vi "CLSUIP_GetControlInformation.vi"(8 "error in (no error)":errorcluster, 11 "Ctl Refnum":refnum<vi>) -> (0 "error out":errorcluster, 2 "Control Information":T1, 3 "Ctl Refnum out":refnum<vi>)   [LabVIEW 2021, in "MemberVICreation.lvlib"]
uses:
  <resource>/Framework/Providers/LVClassLibrary/NewAccessors/MemberVICreation.lvlib
  <resource>/Framework/Providers/LVClassLibrary/NewAccessors/CLSUIP_ControlInformation.ctl
  <vilib>/Utility/miscctls.llb/LVPositionTypeDef.ctl
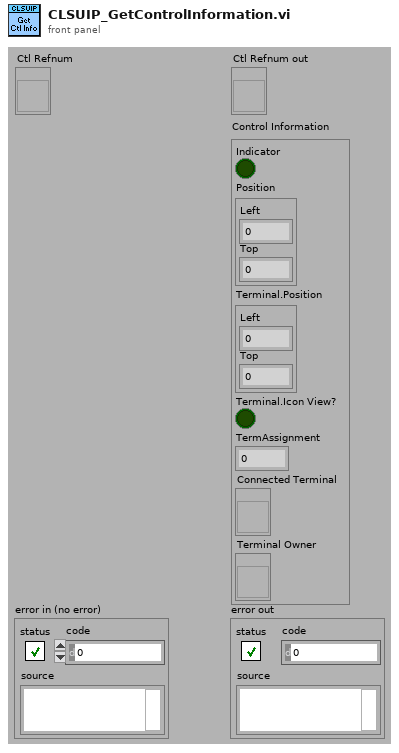
[diagram p1: front panel]
types:
  T1 = typedef "MemberVICreation.lvlib/CLSUIP_ControlInformation.ctl" = cluster{"Indicator":bool, "Position":T2, "Terminal.Position":T2, "Terminal.Icon View?":bool, "TermAssignment":i32, "Connected Terminal":refnum<vi>, "Terminal Owner":refnum<vi>}
  T2 = typedef "LVPositionTypeDef.ctl" = cluster{"Left":i32, "Top":i32}
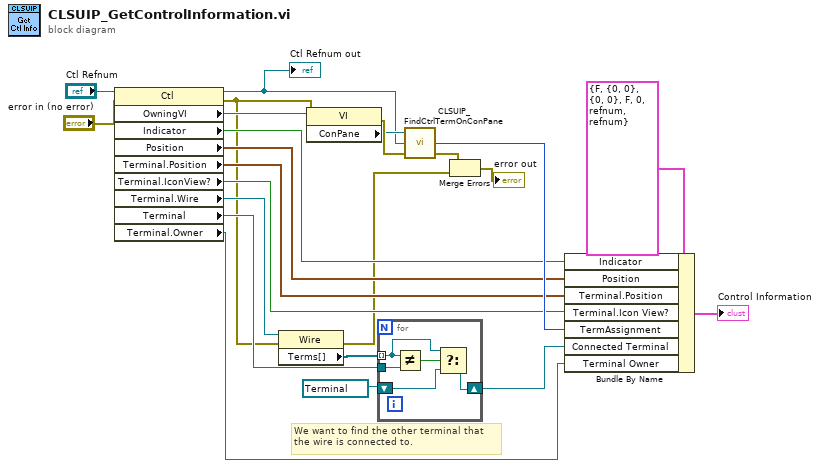
[diagram p0: block diagram]
diagram:
  # "We want to find the other terminal that\nthe wire is connected to."
  n1 = property class="Ctl"(reference="Ctl Refnum", error in="error in (no error)") -> (reference out=w11:refnum<vi>, error out=w5:errorcluster, "OwningVI"=w22:refnum<vi>, "Indicator"=w19:bool, "Position"=w18:T2, "Terminal.Position"=w17:T2, "Terminal.IconView?"=w16:bool, "Terminal.Wire"=w10:refnum<vi>, "Terminal"=w8:refnum<vi>, "Terminal.Owner"=w1:refnum<vi>)
  "Ctl Refnum out" <- w11
  n2 = property class="Wire"(reference=w10, error in=w5) -> (error out=w3:errorcluster, "Terms[]"=w9:refnum<vi>[])  [unwired: 1 out]
  n3 = property class="VI"(reference=w22, error in=w5) -> (error out=w14:errorcluster, "ConPane"=w12:refnum<vi>)  [unwired: 1 out]
  n4 = for {
    tunnel: w9 -> [w24] mode=indexing
    shift-right: [w25] -> w7
    shift-left: refnum<vi> refnum ("Connected Terminal") -> [w26]
    tunnel: w8 -> [w27]
    n5 = Not Equal?(x=w24, y=w27) -> (x != y?=w28:bool)
    n6 = Select(t=w24, s=w28, f=w26) -> (s? t:f=w25:refnum<vi>)
  }
  n7 = call <resource>:"CLSUIP_FindCtrlTermOnConPane.vi"("error in (no error)"=w14, "Ctl Refnum"=w11, "ConPane"=w12) -> ("error out"=w4:errorcluster, "Terminal Index"=w20:i32)  [unwired: 1 out]
  n8 = Merge Errors(w4, w3) -> (→"error out":errorcluster)
  n9 = Bundle By Name(cluster=T1 {"Indicator"=FALSE, "Position"={"Left"=0, "Top"=0}, "Terminal.Position"={"Left"=0, "Top"=0}, "Terminal.Icon View?"=FALSE, "TermAssignment"=0, "Connected Terminal"=refnum, "Terminal Owner"=refnum} ("Control Information"), "Indicator"=w19, "Position"=w18, "Terminal.Position"=w17, "Terminal.Icon View?"=w16, "TermAssignment"=w20, "Connected Terminal"=w7, "Terminal Owner"=w1) -> (→"Control Information":T1)
